vi "servo.vi"() -> ()   [LabVIEW 2013]
uses:
  <vilib>/LabVIEW Interface for Arduino/LabVIEW Interface for Arduino.lvlib
panel:
  in  "Knob":dbl(knob) scale=0.0..180.0
  out "Angle (Degrees) 2":u8(knob)=15 scale=0.0..180.0
  in  "DIO Pin (2)":u8=2
  in  "stop":bool
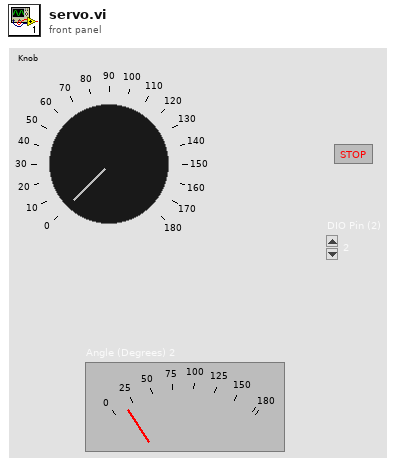
[diagram p1: front panel]
types:
  T1 = typedef "LabVIEW Interface for Arduino.lvlib/Arduino Resource.ctl" = cluster{"VISA resource":refnum<visa-resource-name>, "Board Type":T2, "Connection Type":enum8{"USB / Serial"}, "Bytes Per Packet (15)":u8}
  T2 = typedef "LabVIEW Interface for Arduino.lvlib/Board Type.ctl" = enum16{"Uno", "Dimuelanove w/Atmega 328", "Mega 2560"}
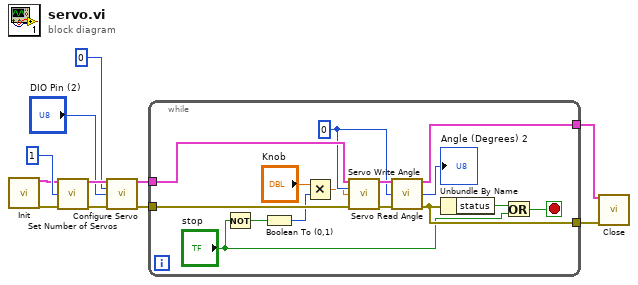
[diagram p0: block diagram]
diagram:
  n1 = call <vilib>:"Init.vi"() -> ("Arduino Resource"=w2:T1, "error out"=w1:errorcluster)  [unwired: 18 in]
  n2 = call <vilib>:"Set Number of Servos.vi"("Arduino Resource"=w2, "Number Of Servos (1)"=u8 1, "error in"=w1) -> ("Arduino Resource"=w10:T1, "error out"=w11:errorcluster)  [unwired: 11 in]
  n3 = call <vilib>:"Configure Servo.vi"("Arduino Resource"=w10, "Servo Number (0)"=u8 0, "DIO Pin (2)"="DIO Pin (2)", "error in"=w11) -> ("Arduino Resource"=w8:T1, "error out"=w9:errorcluster)  [unwired: 10 in]
  n4 = while {
    tunnel: w9 -> [w26]
    tunnel: [w19] -> w3
    tunnel: w8 -> [w25]
    tunnel: [w22] -> w4
    stop <- w23 stop-if-true
    w17 = 0
    n5 = Not(x="stop") -> (.not. x?=w15:bool)
    n6 = Boolean To (0,1)(Boolean=w15) -> (0, 1=w13:i16)
    n7 = Multiply(x="Knob", y=w13) -> (x*y=w12:dbl)
    n8 = call <vilib>:"Servo Write Angle.vi"("Arduino Resource"=w25, "Servo Number"=w17, "Angle (Degrees)"=w12, "error in"=w26) -> ("Arduino Resource"=w21:T1, "error out"=w20:errorcluster)  [unwired: 10 in]
    n9 = call <vilib>:"Servo Read Angle.vi"("Arduino Resource"=w21, "Servo Number"=w17, "error in"=w20) -> ("Arduino Resource"=w22:T1, "Angle (Degrees)"=→"Angle (Degrees) 2":u8, "error out"=w19:errorcluster)  [unwired: 10 in]
    n10 = Unbundle By Name(w19) -> ("status"=w24:bool)
    n11 = Or(x=w24, y="stop") -> (x .or. y?=w23:bool)
  }
  n12 = call <vilib>:"Close.vi"("Arduino Resource"=w4, "error in"=w3) -> ()  [unwired: 13 in, 1 out]
